vi "UV-VIS SetAcquisitionMode.vi"(3 "error in (no error)":errorcluster, 4 "mode":T1=enum."Single Scan", 5 "Control in":refnum<class "CCD_camera.lvclass">) -> (0 "error out":errorcluster, 1 "DLL error code":u32, 2 "Control out":refnum<class "CCD_camera.lvclass">)   [LabVIEW 2020, in "CCD_camera.lvclass"]
doc: "This function will set the acquisition mode to be used on the next <B>StartAcquisition</B>.\n\n<B>Parameter:</B>\nmode - the acquisition mode.\n Valid values: 0,5,7,8 Reserved DO NOT USE\n 1 - Single Scan\n 2 - Accumulate\n 3 - Kinetics\n 4 - Fast Kinetics\n 6 - Frame Transfer\n 9 - Time Delayed Integration (requires special files)\n\n<B>Error codes:</B>\nDRV_SUCCESS - Acquisition mode set.\nDRV_NOT_INITIALIZED - System not initialized.\nDRV_ACQUIRING - Acquisition in progress.\nDRV_P1INVALID - Acquisition Mode invalid.\n\n<B>NOTES:</B>\n<B>In modes 5 and 7 the system uses a \"Run Till Abort\" acquisition mode for non-Frame Transfer and Frame Transfer respectively. In these modes the camera continually acquires data until the AbortAcquisition function is called. These modes have not been tested under all conditions and hence are not listed above. You are free to try them. If you encounter any problem please notify us.</B>"
uses:
  CCD_camera.lvclass
  dependecies/AcquisitionMode_mode typedef.ctl
  C:/dev/TRANCON/Classes/Detector/Detector.lvclass
  Detector.lvclass/Detector.ctl
  Detector.lvclass
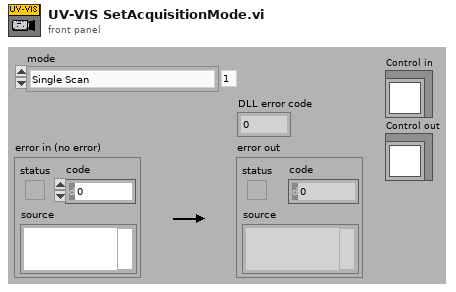
[diagram p1: front panel]
types:
  T1 = typedef "AcquisitionMode_mode typedef.ctl" = enum16{"Reserved (0)", "Single Scan", "Accumulate", "Kinetics", "Fast Kinetics", "Run Till Abort for non-Frame Transfer", "Frame Transfer", "Run Till Abort for Frame Transfer", "Reserved (8)", "Time Delayed Integration"}
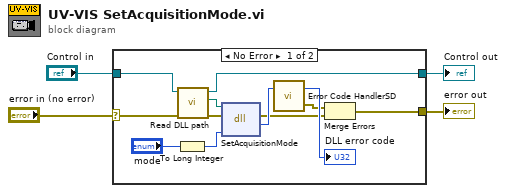
[diagram p0: block diagram]
diagram:
  n1 = case shown="No Error" "error in (no error)" {
    selector: "error in (no error)" -> [w11 w18]
    tunnel: [w6 w18] -> w3
    tunnel: [w5 w17] -> w2
    tunnel: "Control in" -> [w12 w17]
    frame No Error {
      n2 = To Long Integer(number="mode") -> (32bit integer=w14:i32)
      n3 = call "Read DLL path.vi"("error in (no error)"=w11, "Detector in"=w12) -> ("error out"=w9:errorcluster, "DLL path"=w10:path, "Detector out"=w5:refnum<class "CCD_camera.lvclass">)  [unwired: 7 in]
      n4 = dll-call lib="S:/TRANCON/DLL/Atmcd32d.dll" fn="SetAcquisitionMode"(path in=w10, error in=w9, "mode"=w14) -> (error out=w8:errorcluster, "return type"=w16:u32)  [unwired: 2 in, 1 out]
      n5 = call "Error Code HandlerSD.vi"("DLL error code"=w16) -> ("error out"=w7:errorcluster, "dup DLL error code"=→"DLL error code":u32)  [unwired: 1 in]
      n6 = Merge Errors(w7, w8) -> (w6:errorcluster)
    }
    frame Error {
    }
  }
  "error out" <- w3
  "Control out" <- w2
